vi "graph_detailed_info.vi"() -> ()   [LabVIEW 2020]
uses:
  <vilib>/measure/NI_MABase.lvlib
panel:
  in  "sampling info":cluster{"Fs":dbl, "#s":dbl}={"Fs"=1000.0, "#s"=1000.0} {"Fs" format="%.2p"}
  out "dt":dbl format="%#_13g"
  out "Sampling Rate":dbl
  out "Numeric":i32
  out "Waveform Graph":waveform(dbl)(graph)
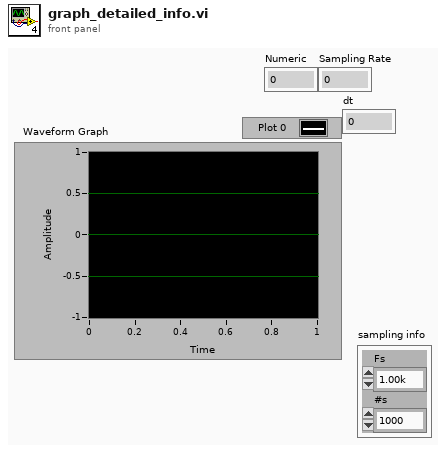
[diagram p1: front panel]
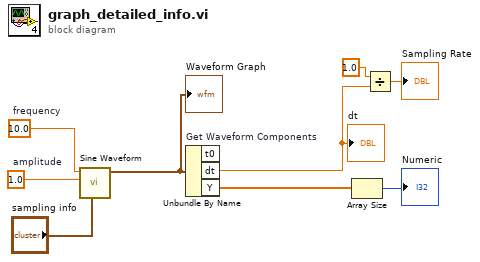
[diagram p0: block diagram]
diagram:
  w8 = 1.0  # amplitude
  w9 = 10.0  # frequency
  n1 = call <vilib>:"Sine Waveform.vi"("sampling info"="sampling info", "amplitude"=w8, "frequency"=w9) -> ("signal out"=w7:waveform(dbl))  [unwired: 7 in, 1 out]
  "Waveform Graph" <- w7
  n2 = Unbundle By Name "Get Waveform Components"(w7) -> ("dt"=w2:dbl, "Y"=w6:dbl[])  [unwired: 1 out]
  "dt" <- w2
  n3 = Array Size(array=w6) -> (size(s)=→"Numeric":i32)
  n4 = Divide(x=1.0, y=w2) -> (x/y=→"Sampling Rate":dbl)
